vi "CalculatePhaseMagnitude_indexed.vi"(7 "IQ indexes":i32[][](array[numeric]), 9 "phase reference channel":i32, 10 "previous phase":dbl[](array[numeric]), 11 "data":dbl[][](array[numeric])) -> (1 "last phase":dbl[](array[numeric]), 2 "Magnitude":dbl[][](array[numeric]), 3 "Phase":dbl[][](array[numeric]))   [LabVIEW 2013]
uses:
  <vilib>/Analysis/NI_AALPro.lvlib
panel:
  # "each row is I and then Q of one channel"
  # "each row is a pair of indexes in the data matrix.\nThe first index is I of that channelm the second is Q of that channel"
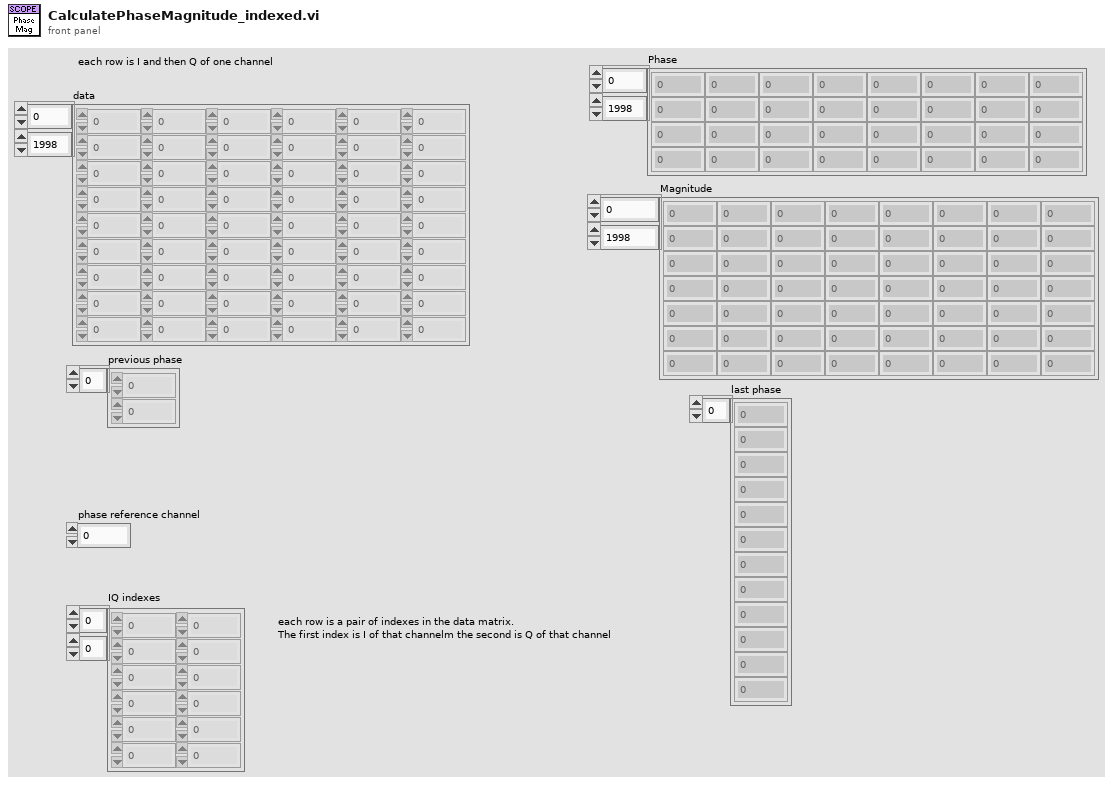
[diagram p1: front panel]
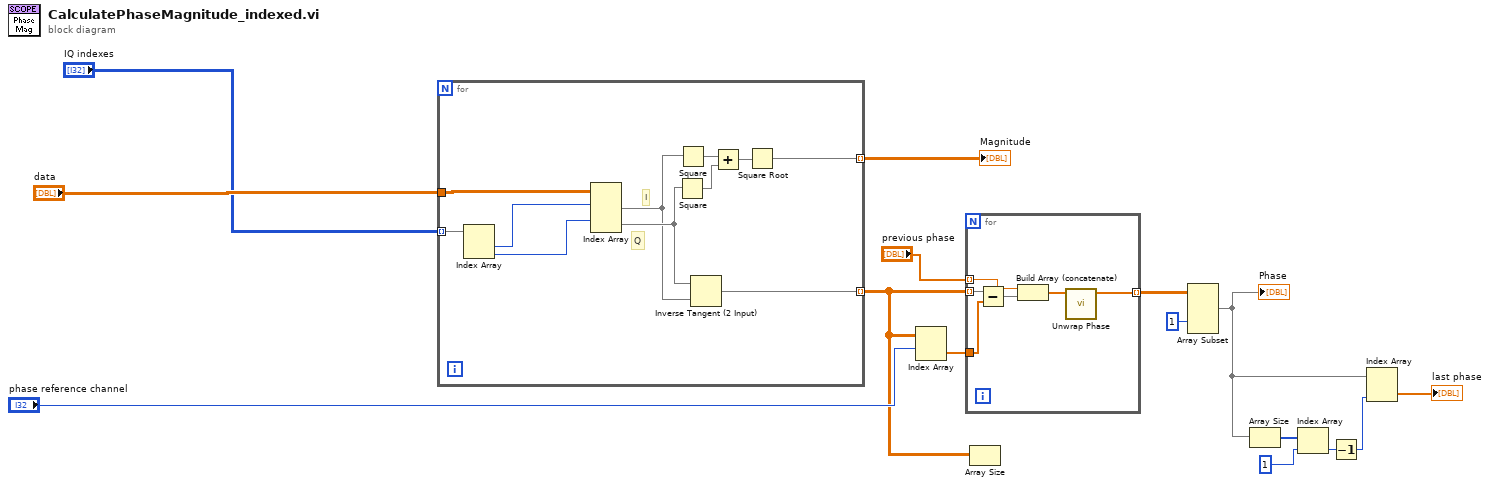
[diagram p0: block diagram]
diagram:
  n1 = for {
    tunnel: "data" -> [w26]
    tunnel: [w20] -> w14 mode=indexing
    tunnel: [w19] -> w2 mode=indexing
    tunnel: "IQ indexes" -> [w18] mode=indexing
    # "Q"
    # "I"
    n2 = Index Array(array=w18) -> (element #1=w17:i32, element #2=w16:i32)  [unwired: 2 in]
    n3 = Index Array(array=w26, index (row) #1=w17, index (row) #2=w16) -> (element #1=w21:dbl[], element #2=w22:dbl[])  [unwired: 2 in]
    n4 = Square(x=w22) -> (x^2=w24:dbl[])
    n5 = Square(x=w21) -> (x^2=w25:dbl[])
    n6 = Inverse Tangent (2 Input)(1:w21, 2:w22) -> (0:w19:dbl[])
    n7 = Add(x=w25, y=w24) -> (x+y=w23:dbl[])
    n8 = Square Root(x=w23) -> (sqrt(x)=w20:dbl[])
  }
  "Magnitude" <- w14
  n9 = Index Array(array=w2, index (row)="phase reference channel") -> (element=w12:dbl[])  [unwired: 1 in]
  n10 = for {
    tunnel: w2 -> [w32] mode=indexing
    tunnel: w12 -> [w31]
    tunnel: [w30] -> w8 mode=indexing
    tunnel: "previous phase" -> [w28] mode=indexing
    n11 = Subtract(x=w32, y=w31) -> (x-y=w29:dbl[])
    n12 = Build Array (concatenate)(w28, w29) -> (w27:dbl[])
    n13 = call <vilib>:"Unwrap Phase.vi"("Phase"=w27) -> ("Unwrapped Phase"=w30:dbl[])  [unwired: 9 in, 1 out]
  }
  n14 = Array Size(array=w2) -> ()  [unwired: 1 out]
  n15 = Array Subset(array=w8, index (col)=1 ("index")) -> (w3:dbl[][])  [unwired: 3 in]
  "Phase" <- w3
  n16 = Array Size(array=w3) -> (size(s)=w9:i32[])
  n17 = Index Array(array=w9, index=1) -> (element=w7:i32)
  n18 = Decrement(x=w7) -> (x-1=w5:i32)
  n19 = Index Array(array=w3, index (col)=w5) -> (element=→"last phase":dbl[])  [unwired: 1 in]
